vi "daqio_Get_Device_Events.vi"(8 "error in (no error)":errorcluster, 11 "daq.io type in":T2={"daq.io ref"=refnum, "daq.io API Base"="http://dashboard.daq.io/api/v1", "Device Key"="", "Account ID"="", "online"=TRUE, "SSL"=TRUE, "buffer"=TRUE}) -> (0 "error out":errorcluster, 2 "All Events":T1[](array[typedef]), 3 "daq.io type out":T2={"daq.io ref"=refnum, "daq.io API Base"="http://dashboard.daq.io/api/v1", "Device Key"="", "Account ID"="", "online"=TRUE, "SSL"=TRUE, "buffer"=TRUE})   [LabVIEW 2013, in "daqio minimal.lvlib"]
doc: "This VI returns all Events that occured for a specific Device."
uses:
  daqio minimal.lvlib
  _typedefs/daqio-Type.ctl
  <vilib>/httpClient/ClientHandle.ctl
  _typedefs/daqio-Event.ctl
  <vilib>/Easy HTTP Client/Easy HTTP.lvlib
  <vilib>/httpClient/LabVIEWHTTPClient.lvlib
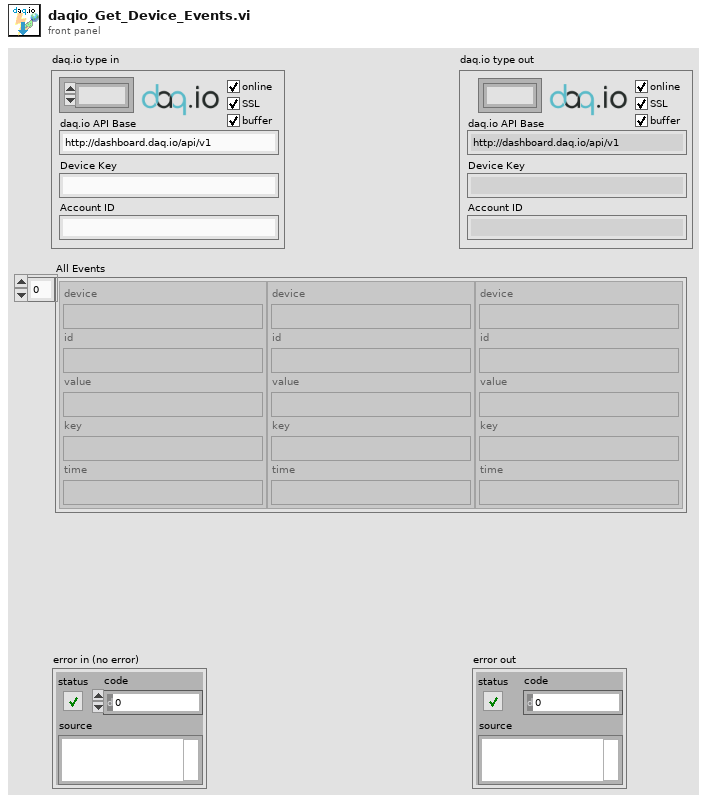
[diagram p1: front panel]
types:
  T1 = typedef "daqio minimal.lvlib/daqio-Event.ctl" = cluster{"device":string, "id":string, "value":string, "key":string, "time":string}
  T2 = typedef "daqio minimal.lvlib/daqio-Type.ctl" = cluster{"daq.io ref":T3, "daq.io API Base":string, "Device Key":string, "Account ID":string, "online":bool, "SSL":bool, "buffer":bool}
  T3 = typedef "LabVIEWHTTPClient.lvlib/ClientHandle.ctl" = refnum<k1>
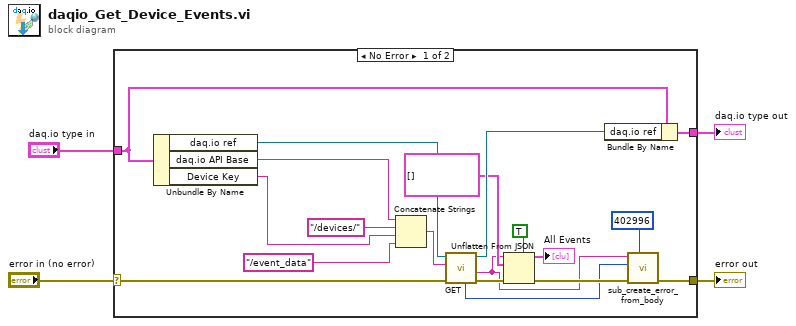
[diagram p0: block diagram]
diagram:
  n1 = case shown="No Error" "error in (no error)" {
    selector: "error in (no error)" -> [w19 w24]
    tunnel: "daq.io type in" -> [w23 w25]
    tunnel: [w22 w25] -> w3
    tunnel: [w13 w24] -> w2
    frame No Error {
      n2 = Unbundle By Name(w23) -> ("daq.io ref"=w21:T3, "daq.io API Base"=w7:string, "Device Key"=w5:string)
      n3 = Concatenate Strings(w7, "/devices/" ("string"), w5, "/event_data") -> (w17:string)
      n4 = call <vilib>:"GET.vi"("error in (no error)"=w19, "url"=w17, "client handle"=w21) -> ("error out"=w18:errorcluster, "body"=w11:string, "client handle out"=w20:T3, "HTTP Response Code"=w12:i32)  [unwired: 4 in, 1 out]
      n5 = Unflatten From JSON(enable LabVIEW extensions? (T)=TRUE, JSON string=w11, type and defaults=T1[] [], error in (no error)=w18) -> (value=→"All Events":T1[], error out=w14:errorcluster)  [unwired: 3 in]
      n6 = Bundle By Name(cluster=w23, "daq.io ref"=w20) -> (w22:T2)
      n7 = call "sub_create_error_from_body.vi"("error code"=402996, "error in (no error)"=w14, "http code"=w12, "body"=w11) -> ("error out"=w13:errorcluster)  [unwired: 7 in]
    }
    frame Error {
    }
  }
  "error out" <- w2
  "daq.io type out" <- w3
